vi "Z Aux Direct M Eclipse.vi"(0 "handle":u32, 1 "fcenter2":sgl, 2 "fADis":sgl, 5 "fend1":sgl, 7 "fend2":sgl, 9 "fcenter1":sgl, 11 "error in (no error)":errorcluster caption="错误输入（无错误）", 12 "idirection":i32, 13 "fBDis":sgl) -> (4 "handle out":u32, 6 "function return":i32, 15 "error out":errorcluster caption="错误输出")   [LabVIEW 2015, in "zauxdll.lvlib"]
doc: "int32 __stdcall ZAux_Direct_MEclipse(ZMC_HANDLE handle, float fend1, float fend2, float fcenter1, float fcenter2, int idirection, float fADis, float fBDis);"
uses:
  zauxdll.lvlib
  zauxdll.dll
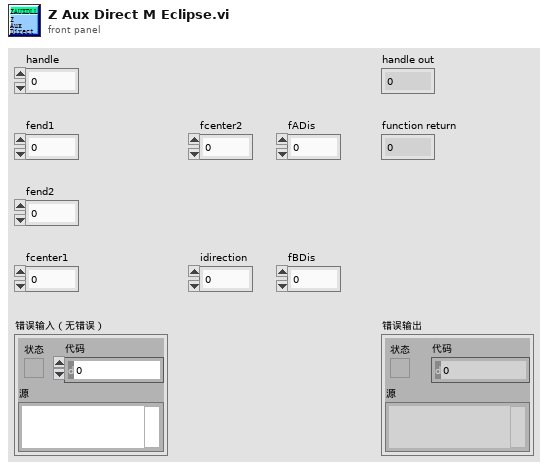
[diagram p1: front panel]
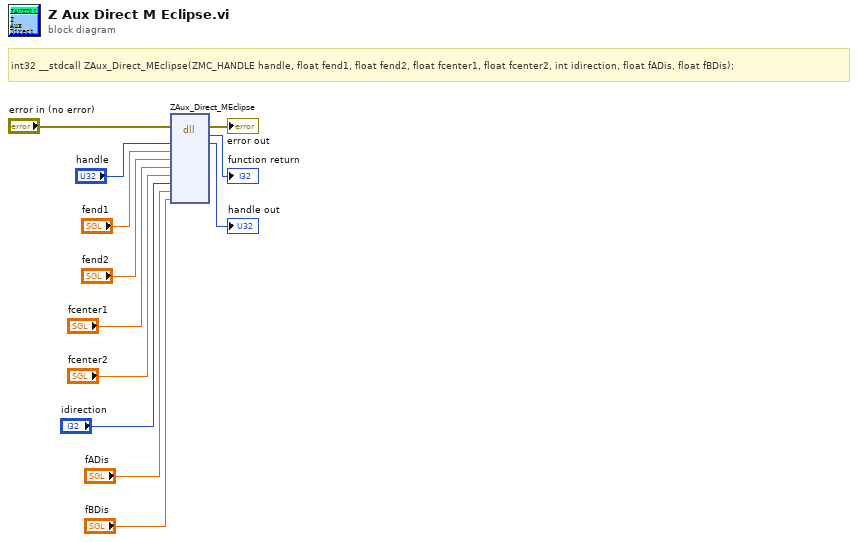
[diagram p0: block diagram]
diagram:
  # "int32 __stdcall ZAux_Direct_MEclipse(ZMC_HANDLE handle, float fend1, float fend2, float fcenter1, float fcenter2, int idirection, float fADis, float fBDis);"
  n1 = dll-call lib="C:/Users/VIC/Desktop/GOGORO_Oringnal - Panasonic/system/LLB/zmotion/zaux/zauxdll.*" fn="ZAux_Direct_MEclipse"(error in="error in (no error)", "handle"="handle", "fend1"="fend1", "fend2"="fend2", "fcenter1"="fcenter1", "fcenter2"="fcenter2", "idirection"="idirection", "fADis"="fADis", "fBDis"="fBDis") -> (error out=→"error out":errorcluster, →"function return":i32, "handle"=→"handle out":u32)  [unwired: 9 in, 1 out]
